vi "Tree_AssertAllTags_Tests.vi"(11 "error in":errorcluster) -> (15 "error out":errorcluster)   [LabVIEW 2016, in "DronaTest.lvlib"]
uses:
  DronaTest.lvlib
  APIs/Stimulus/ControlValue/SetValueAuto.vi
  APIs/Assert/AssertControlValue/Controls/Tree/AssertAllTags.vi
  <vilib>/addons/_JKI Toolkits/Caraya/classes/Assert/Assert Error.vi
  <vilib>/addons/_JKI Toolkits/Caraya/classes/Assert/Assert Equal Value_Variant.vi
  <vilib>/addons/_JKI Toolkits/Caraya/classes/Test/Test.lvclass
  Drona.lvlib
  <vilib>/SLL Toolkit/SLL Debug/SLL Debug.lvlib
  <vilib>/addons/_JKI Toolkits/Caraya/classes/Assert/Assert.lvclass
  APIs/Stimulus/ControlValue/ControlValue.lvlib
  APIs/Assert/AssertControlValue/Controls/Tree/AssertTree.lvlib
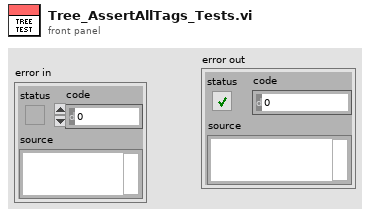
[diagram p1: front panel]
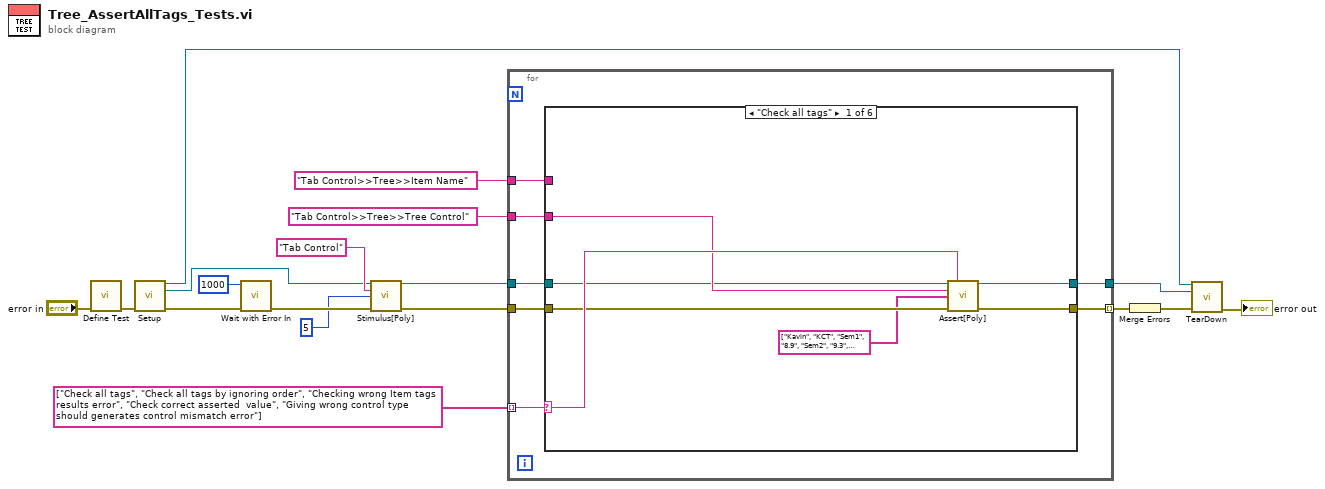
[diagram p0: block diagram]
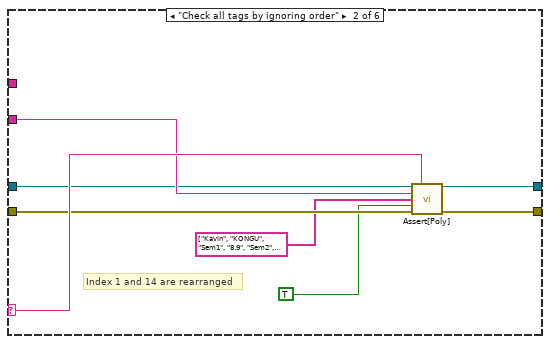
[diagram p2: hidden frame]
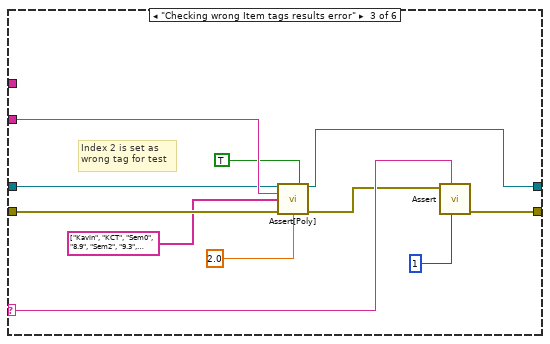
[diagram p3: hidden frame]
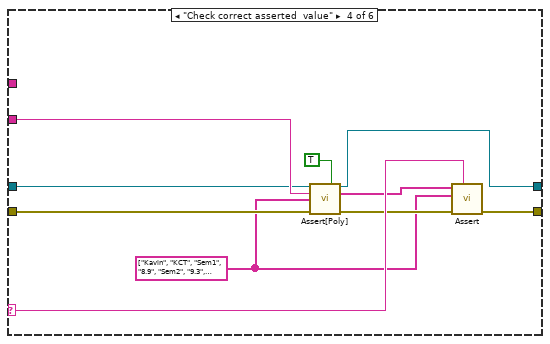
[diagram p4: hidden frame]
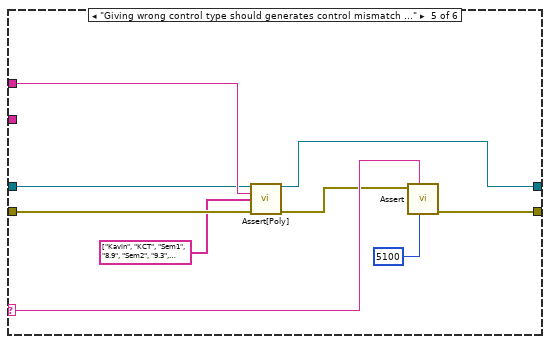
[diagram p5: hidden frame]
diagram:
  n1 = call <vilib>:"Define Test.vi"("error in (no error)"="error in") -> ("error out"=w9:errorcluster)  [unwired: 10 in]
  n2 = call "Setup.vi"("error in (no error)"=w9) -> ("Application Ref"=w5:refnum<vi>, "VI out"=w7:refnum<vi>, "error out"=w8:errorcluster)  [unwired: 12 in]
  n3 = call <vilib>:"Wait with Error In.vi"("error in (no error)"=w8, "milliseconds to wait"=u32 1000) -> ("error out"=w16:errorcluster)  [unwired: 9 in]
  n4 = call-poly "Stimulus[Poly].vi"("VI Reference In"=w7, "Control Path"="Tab Control", "Value (Signaling)"=5, "error in"=w16) -> ("VI Reference Out"=w12:refnum<vi>, "error out"=w15:errorcluster)  [unwired: 10 in]
  n5 = for {
    tunnel: w12 -> [w24]
    tunnel: "Tab Control>>Tree>>Tree Control" ("Control Path") -> [w23]
    tunnel: "Tab Control>>Tree>>Item Name" ("Control Path") -> [w22]
    tunnel: string[] ["Check all tags", "Check all tags by ignoring order", "Checking wrong Item tags results error", "Check correct asserted  value", "Giving wrong control type should generates control mismatch error"] -> [w20] mode=indexing
    tunnel: [w19] -> w4
    tunnel: w15 -> [w25]
    tunnel: [w21] -> w10 mode=indexing
    n6 = case shown="\"Check all tags\"" w20 {
      selector: w20 -> [w30 w38 w50 w60 w69 _]
      tunnel: w25 -> [w28 w36 w43 w56 w64 w72]
      tunnel: w24 -> [w27 w35 w42 w55 w63 w71]
      tunnel: w23 -> [w29 w37 w48 w59 _ _]
      tunnel: w22 -> [_ _ _ _ w66 _]
      tunnel: [w32 w40 w51 w61 w70 w72] -> w21
      tunnel: [w31 w39 w47 w58 w65 w71] -> w19
      frame "Check all tags" {
        n7 = call-poly "Assert[Poly].vi"("VI Reference In"=w27, "Test Label"=w30, "Control Path"=w29, "Item Tags"=string[] ["Kavin", "KCT", "Sem1", "8.9", "Sem2", "9.3", "Sem3", "9.3_1", "Sem4", "9.5", "Sem5", "9.2", "Sem6", "9.1", "KONGU", "Sem1_1", "8.8", "Sem2_1", "9.5_1", "Sem3_1", "9.6", "Sem4_1", "9.6_1", "Sem5_1", "9.4", "Sem6_1", "9.7"] ("All Tags"), "Error In"=w28) -> ("VI Reference Out"=w31:refnum<vi>, "Error Out"=w32:errorcluster)  [unwired: 8 in, 1 out]
      }
      frame "Check all tags by ignoring order" {
        # "Index 1 and 14 are rearranged"
        n8 = call-poly "Assert[Poly].vi"("VI Reference In"=w35, "Test Label"=w38, "Control Path"=w37, "Item Tags"=string[] ["Kavin", "KONGU", "Sem1", "8.9", "Sem2", "9.3", "Sem3", "9.3_1", "Sem4", "9.5", "Sem5", "9.2", "Sem6", "9.1", "KCT", "Sem1_1", "8.8", "Sem2_1", "9.5_1", "Sem3_1", "9.6", "Sem4_1", "9.6_1", "Sem5_1", "9.4", "Sem6_1", "9.7"] ("All Tags"), "Ignore Order? (F)"=TRUE, "Error In"=w36) -> ("VI Reference Out"=w39:refnum<vi>, "Error Out"=w40:errorcluster)  [unwired: 7 in, 1 out]
      }
      frame "Checking wrong Item tags results error" {
        # "Index 2 is set as \nwrong tag for test"
        n9 = call-poly "Assert[Poly].vi"("VI Reference In"=w42, "Assert Only? (F)"=TRUE, "Control Path"=w48, "Item Tags"=string[] ["Kavin", "KCT", "Sem0", "8.9", "Sem2", "9.3", "Sem3", "9.3_1", "Sem4", "9.5", "Sem5", "9.2", "Sem6", "9.1", "KONGU", "Sem1_1", "8.8", "Sem2_1", "9.5_1", "Sem3_1", "9.6", "Sem4_1", "9.6_1", "Sem5_1", "9.4", "Sem6_1", "9.7"] ("All Tags"), "Error In"=w43, "Timeout(5 sec)"=2.0) -> ("VI Reference Out"=w47:refnum<vi>, "Error Out"=w46:errorcluster)  [unwired: 7 in, 1 out]
        n10 = call-poly <vilib>:"Assert.vi"("error code (1)"=1, "Label"=w50, "Error?"=w46) -> ("error out"=w51:errorcluster)  [unwired: 8 in]
      }
      frame "Check correct asserted  value" {
        w52 = string[] ["Kavin", "KCT", "Sem1", "8.9", "Sem2", "9.3", "Sem3", "9.3_1", "Sem4", "9.5", "Sem5", "9.2", "Sem6", "9.1", "KONGU", "Sem1_1", "8.8", "Sem2_1", "9.5_1", "Sem3_1", "9.6", "Sem4_1", "9.6_1", "Sem5_1", "9.4", "Sem6_1", "9.7"] ("All Tags")
        n11 = call-poly "Assert[Poly].vi"("VI Reference In"=w55, "Assert Only? (F)"=TRUE, "Control Path"=w59, "Item Tags"=w52, "Error In"=w56) -> ("VI Reference Out"=w58:refnum<vi>, "Asserted Value"=w53:string[], "Error Out"=w54:errorcluster)  [unwired: 8 in]
        n12 = call-poly <vilib>:"Assert.vi"("Label"=w60, "error in (no error)"=w54, "Y"=w52, "X"=w53) -> ("error out"=w61:errorcluster)  [unwired: 7 in]
      }
      frame "Giving wrong control type should generates control mismatch error" {
        n13 = call-poly "Assert[Poly].vi"("VI Reference In"=w63, "Control Path"=w66, "Item Tags"=string[] ["Kavin", "KCT", "Sem1", "8.9", "Sem2", "9.3", "Sem3", "9.3_1", "Sem4", "9.5", "Sem5", "9.2", "Sem6", "9.1", "KONGU", "Sem1_1", "8.8", "Sem2_1", "9.5_1", "Sem3_1", "9.6", "Sem4_1", "9.6_1", "Sem5_1", "9.4", "Sem6_1", "9.7"] ("All Tags"), "Error In"=w64) -> ("VI Reference Out"=w65:refnum<vi>, "Error Out"=w67:errorcluster)  [unwired: 9 in, 1 out]
        n14 = call-poly <vilib>:"Assert.vi"("error code (1)"=5100, "Label"=w69, "Error?"=w67) -> ("error out"=w70:errorcluster)  [unwired: 8 in]
      }
      frame Default {
      }
    }
  }
  n15 = Merge Errors(w10) -> (w6:errorcluster)
  n16 = call "TearDown.vi"("Application Ref"=w5, "VI in"=w4, "error in (no error)"=w6) -> ("error out"=→"error out":errorcluster)  [unwired: 12 in]
